vi "Parse Configuration String.vi"(8 "error in (no error)":errorcluster, 10 "Configuration String Lines":string[](array[string]), 11 "Configuration In":T1={"dirty"=FALSE, "path"=path "", "Fileopts"={"Name/Value delimiter (\"=\")"="=", "Comment delimiter (\";\")"=";"}, "Section Lookup"=variant, "Key Lookup"=variant, "Raw File"=[]}) -> (0 "error out":errorcluster, 3 "Configuration Out":T1={"dirty"=FALSE, "path"=path "", "Fileopts"={"Name/Value delimiter (\"=\")"="=", "Comment delimiter (\";\")"=";"}, "Section Lookup"=variant, "Key Lookup"=variant, "Raw File"=[]})   [LabVIEW 2012, in "configlib.lvlib"]
uses:
  configlib.lvlib
  Configuration File Definition.ctl
  File Options.ctl
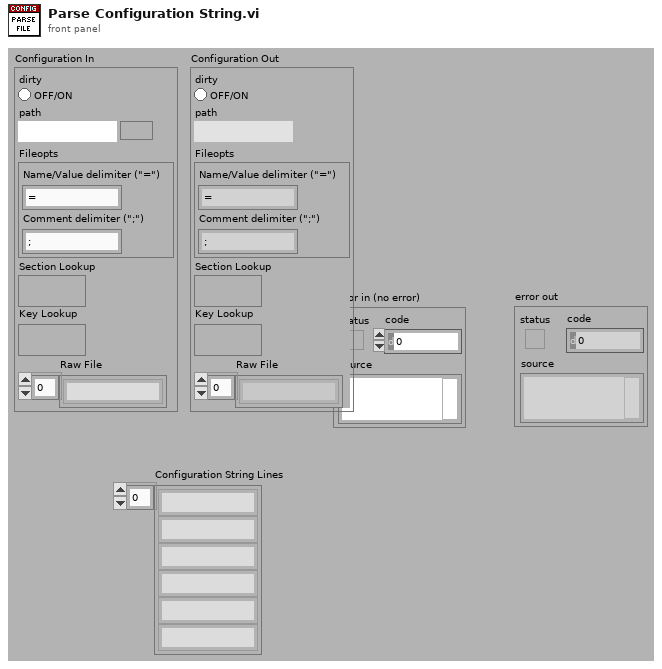
[diagram p1: front panel]
types:
  T1 = typedef "configlib.lvlib/Configuration File Definition.ctl" = cluster{"dirty":bool, "path":path, "Fileopts":T2, "Section Lookup":variant, "Key Lookup":variant, "Raw File":string[]}
  T2 = typedef "configlib.lvlib/File Options.ctl" = cluster{"Name/Value delimiter (\"=\")":string, "Comment delimiter (\";\")":string}
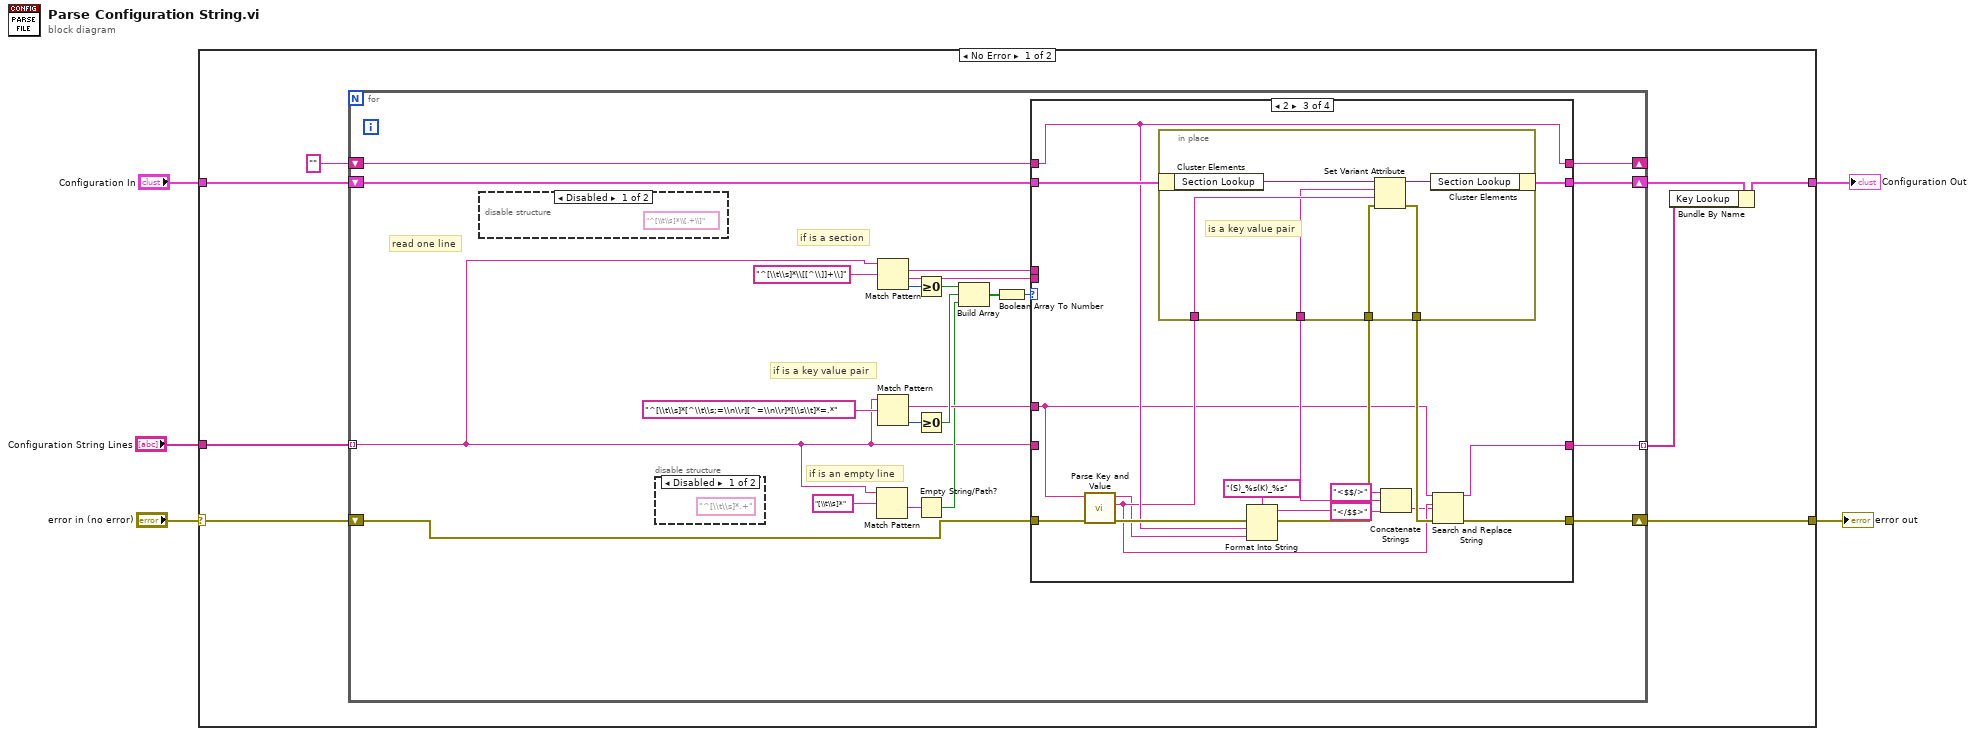
[diagram p0: block diagram]
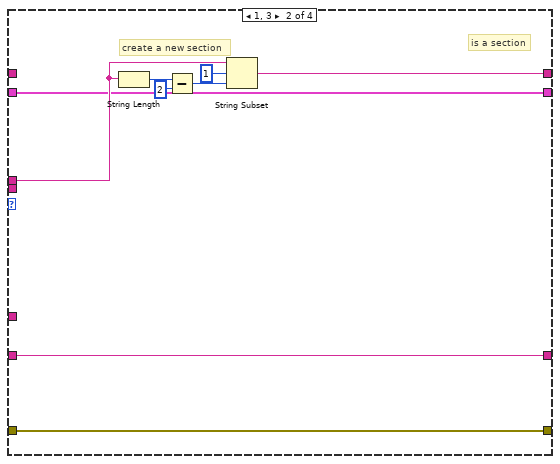
[diagram p5: hidden frame]
diagram:
  n1 = case shown="No Error" "error in (no error)" {
    selector: "error in (no error)" -> [w13 w77]
    tunnel: "Configuration String Lines" -> [w9 _]
    tunnel: [w12 w77] -> w4
    tunnel: "Configuration In" -> [w11 w76]
    tunnel: [w7 w76] -> w2
    frame No Error {
      n2 = for {
        shift-right: [w26] -> w12
        shift-left: w13 -> [w23]
        shift-right: [w19] -> w10
        shift-left: w11 -> [w18]
        shift-right: [w17] -> _
        shift-left: "" -> [w16]
        tunnel: w9 -> [w15] mode=indexing
        tunnel: [w14] -> w6 mode=indexing
        # "if is an empty line"
        # "if is a key value pair"
        # "if is a section"
        # "read one line"
        n3 = disable-structure shown="Disabled" {
          frame Disabled {
            (unwired) "^[\\t\\s]*\\[.+\\]" ("regular expression")
          }
          frame Enabled {
          }
        }
        n4 = disable-structure shown="Disabled" {
          frame Disabled {
            (unwired) "^[\\t\\s]*.+" ("regular expression")
          }
          frame Enabled {
          }
        }
        n5 = Match Pattern(string=w15, regular expression="[\\t\\s]*") -> (after substring=w25:string)  [unwired: 1 in, 3 out]
        n6 = Match Pattern(string=w15, regular expression="^[\\t\\s]*\\[[^\\]]+\\]") -> (match substring=w30:string, after substring=w28:string, offset past match=w35:i32)  [unwired: 1 in, 1 out]
        n7 = Match Pattern(string=w15, regular expression="^[\\t\\s]*[^\\t\\s;=\\n\\r][^=\\n\\r]*[\\s\\t]*=.*") -> (match substring=w29:string, offset past match=w22:i32)  [unwired: 1 in, 2 out]
        n8 = Greater Or Equal To 0?(x=w35) -> (x >= 0?=w34:bool)
        n9 = Greater Or Equal To 0?(x=w22) -> (x >= 0?=w33:bool)
        n10 = Empty String/Path?(string/path=w25) -> (empty?=w27:bool)
        n11 = Build Array(w34, w33, w27) -> (w32:bool[])
        n12 = Boolean Array To Number(Boolean array=w32) -> (number=w31:u32)
        n13 = case shown="2" w31 {
          tunnel: w30 -> [_ w43 _ _]
          tunnel: w29 -> [_ _ w50 _]
          tunnel: w28 -> [_ _ _ _]
          tunnel: w23 -> [w39 w44 w65 w75]
          tunnel: [w39 w44 w52 w75] -> w26
          tunnel: [w38 w42 w63 w74] -> w19
          tunnel: w18 -> [w38 w42 w64 w74]
          tunnel: w15 -> [w36 w40 _ w72]
          tunnel: [w36 w40 w49 w72] -> w14
          tunnel: [w37 w41 w60 w73] -> w17
          tunnel: w16 -> [w37 _ w60 w73]
          frame 0, Default {
            # "by default, it is a comment, \njust add it to kvc"
          }
          frame 1, 3 {
            # "is a section"
            # "create a new section"
            n14 = String Length(string=w43) -> (length=w46:i32)
            n15 = Subtract(x=w46, y=2) -> (x-y=w47:i32)
            n16 = String Subset(string=w43, offset (0)=1, length (rest)=w47) -> (substring=w41:string)
          }
          frame 2 {
            n17 = call "Parse Key and Value.vi"("error in (no error)"=w65, "key value pair"=w50) -> ("error out"=w62:errorcluster, "Value"=w57:string, "Key"=w51:string)  [unwired: 5 in, 2 out]
            n18 = Format Into String(format string="(S)_%s(K)_%s", error in=w62, w60, w51) -> (resulting string=w56:string, error out=w59:errorcluster)  [unwired: 1 in]
            n19 = in-place {
              in-place-border: w57 -> [w71]
              in-place-border: [w70] -> w58
              in-place-border: w56 -> [w69]
              in-place-border: w59 -> [w67]
              # "is a key value pair"
              n20 = in-place-cluster #1(w64) -> ("Section Lookup"=w68:variant)
              n21 = Set Variant Attribute(Variant=w68, name=w69, value=w71, error in=w67) -> (Variant out=w66:variant, error out=w70:errorcluster)  [unwired: 1 out]
              n22 = in-place-cluster #1("Section Lookup"=w66) -> (w63:T1)
            }
            n23 = Concatenate Strings("<$$/>" ("string"), w56, "</$$>" ("string")) -> (w55:string)
            n24 = Search and Replace String(input string=w50, search string=w57, replace string=w55, error in=w58) -> (result string=w49:string, error out=w52:errorcluster)  [unwired: 4 in, 2 out]
          }
          frame 4 {
            # "empty line"
          }
        }
      }
      n25 = Bundle By Name(cluster=w10, "Key Lookup"=w6) -> (w7:T1)
    }
    frame Error {
    }
  }
  "error out" <- w4
  "Configuration Out" <- w2
